vi "Pre Launch Init.vi"(11 "Machine Interface Actor in":refnum<class "Machine Interface.lvclass">) -> (0 "error out":errorcluster, 3 "Machine Interface Actor out":refnum<class "Machine Interface.lvclass">)   [LabVIEW 2019, in "Machine Interface.lvclass"]
doc: "(<B>Filename</B>: Actor Framework.lvlib:Actor.lvclass:Pre Launch Init.vi)\n\nDefines behavior that occurs after the Launch Nested Actor method is invoked but before the actor's Actor Core method begins running.\n\nBy default, this method does nothing. A descendant class may override it to define behavior."
uses:
  Machine Interface.lvclass
  <vilib>/ActorFramework/Actor/Actor.lvclass
panel:
  in  "Trigger Light Camera Sequence":T1
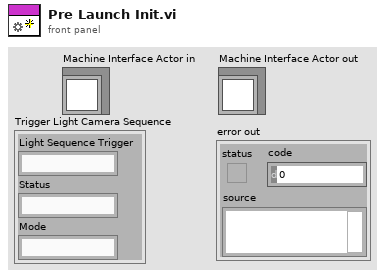
[diagram p1: front panel]
types:
  T1 = cluster{"Light Sequence Trigger":string, "Status":string, "Mode":string}
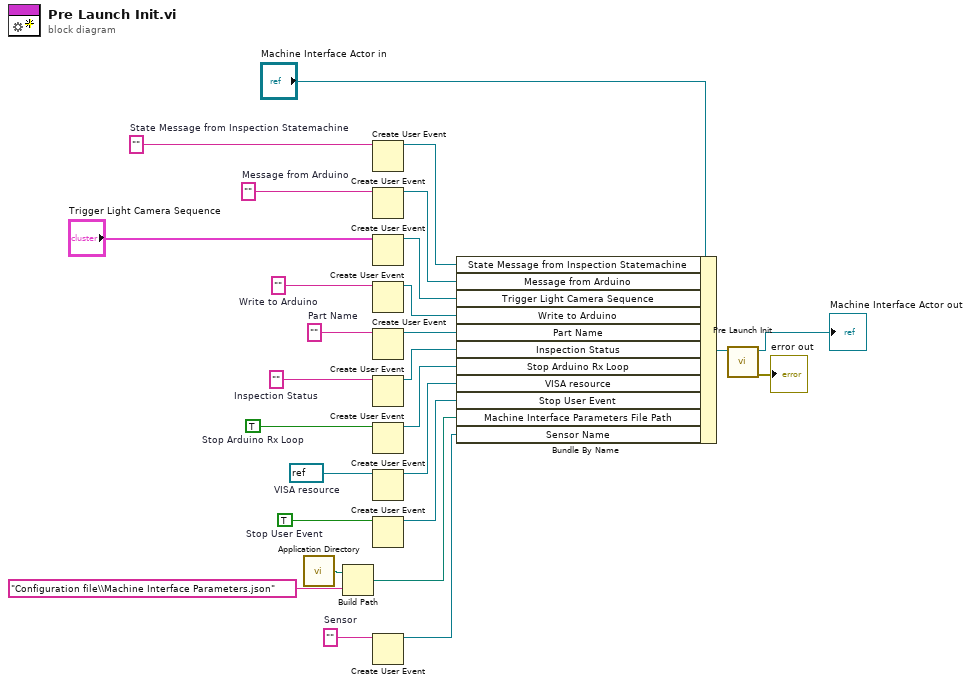
[diagram p0: block diagram]
diagram:
  w3 = ""  # Sensor
  w8 = TRUE  # Stop User Event
  w10 = refnum<visa-resource-name> refnum  # VISA resource
  w19 = ""  # Inspection Status
  w20 = ""  # Part Name
  w21 = ""  # Write to Arduino
  w23 = TRUE  # Stop Arduino Rx Loop
  w24 = ""  # Message from Arduino
  w25 = ""  # State Message from Inspection Statemachine
  n1 = call <vilib>:"Application Directory.vi"() -> ("Application Directory"=w6:path)
  n2 = Build Path(base path=w6, name or relative path="Configuration file\\Machine Interface Parameters.json") -> (appended path=w4:path)
  n3 = Create User Event(user event datatype=w25) -> (user event=w16:refnum<user-event>)  [unwired: 1 in, 1 out]
  n4 = Create User Event(user event datatype=w24) -> (user event=w15:refnum<user-event>)  [unwired: 1 in, 1 out]
  n5 = Create User Event(user event datatype="Trigger Light Camera Sequence") -> (user event=w1:refnum<user-event>)  [unwired: 1 in, 1 out]
  n6 = Create User Event(user event datatype=w21) -> (user event=w14:refnum<user-event>)  [unwired: 1 in, 1 out]
  n7 = Create User Event(user event datatype=w20) -> (user event=w11:refnum<user-event>)  [unwired: 1 in, 1 out]
  n8 = Create User Event(user event datatype=w19) -> (user event=w12:refnum<user-event>)  [unwired: 1 in, 1 out]
  n9 = Create User Event(user event datatype=w23) -> (user event=w13:refnum<user-event>)  [unwired: 1 in, 1 out]
  n10 = Create User Event(user event datatype=w10) -> (user event=w9:refnum<user-event>)  [unwired: 1 in, 1 out]
  n11 = Create User Event(user event datatype=w8) -> (user event=w7:refnum<user-event>)  [unwired: 1 in, 1 out]
  n12 = Create User Event(user event datatype=w3) -> (user event=w2:refnum<user-event>)  [unwired: 1 in, 1 out]
  n13 = Bundle By Name(cluster="Machine Interface Actor in", "State Message from Inspection Statemachine"=w16, "Message from Arduino"=w15, "Trigger Light Camera Sequence"=w1, "Write to Arduino"=w14, "Part Name"=w11, "Inspection Status"=w12, "Stop Arduino Rx Loop"=w13, "VISA resource"=w9, "Stop User Event"=w7, "Machine Interface Parameters File Path"=w4, "Sensor Name"=w2) -> (w17:refnum<class "Machine Interface.lvclass">)
  n14 = call-parent "Pre Launch Init.vi"("Actor in"=w17) -> ("error out"=→"error out":errorcluster, "Actor out"=→"Machine Interface Actor out":refnum<class "Machine Interface.lvclass">)  [unwired: 9 in]
